vi "Configure Module.vi"(8 "error in (no error)":errorcluster, 10 "IOV ref in":refnum<k21>, 11 "Module Template in":refnum<class "9203.lvclass">) -> (0 "error out":errorcluster, 2 "IOV ref out":refnum<k21>, 3 "Module Template out":refnum<class "9203.lvclass">)   [LabVIEW 2011, in "Modules.lvlib" / "9203.lvclass"]
uses:
  9203.lvclass
  9203.lvclass/9203.ctl
  Program Files (x86)/National Instruments/LabVIEW 2011/resource/objmgr/cRIO.rc
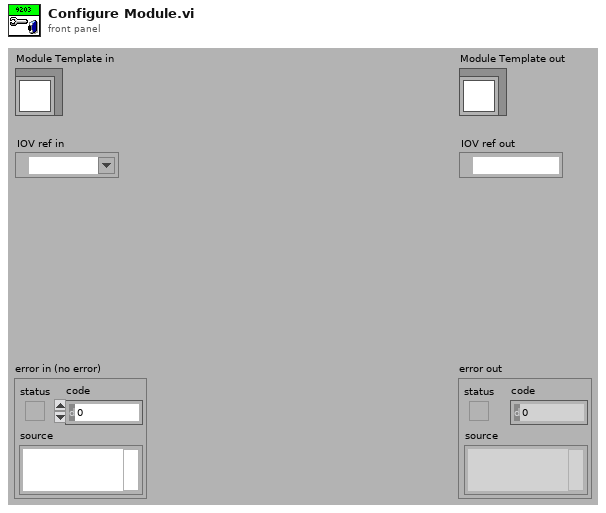
[diagram p1: front panel]
types:
  T1 = typedef "Modules.lvlib/9203.lvclass/Channel Settings.ctl" = cluster{"Range":T2}[]
  T2 = typedef "Modules.lvlib/9203.lvclass/Range.ctl" = u32
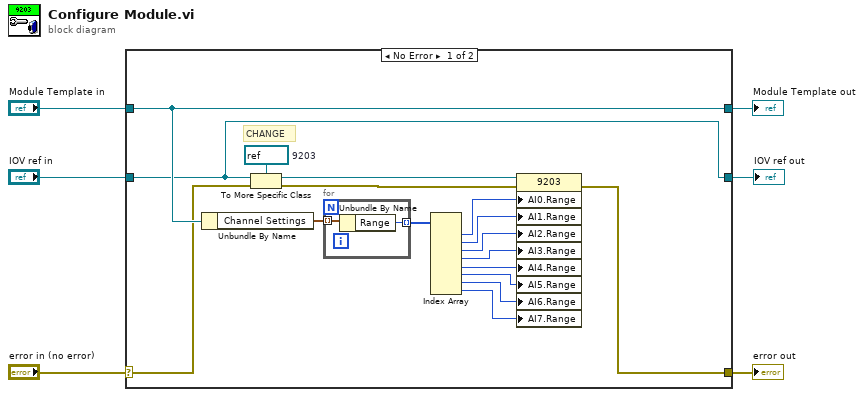
[diagram p0: block diagram]
diagram:
  n1 = case shown="No Error" "error in (no error)" {
    selector: "error in (no error)" -> [w22 w28]
    tunnel: [w18 w28] -> w5
    tunnel: [w23 w27] -> w3
    tunnel: "Module Template in" -> [w23 w27]
    tunnel: "IOV ref in" -> [w17 w26]
    tunnel: [w17 w26] -> w1
    frame No Error {
      w21 = refnum<k21> refnum  # 9203
      # "CHANGE"
      n2 = Unbundle By Name(w23) -> ("Channel Settings"=w16:T1)
      n3 = To More Specific Class(target class=w21, reference=w17, error in=w22) -> (specific class reference=w20:refnum<k21>, error out=w19:errorcluster)
      n4 = for {
        tunnel: w16 -> [w25] mode=indexing
        tunnel: [w24] -> w15 mode=indexing
        n5 = Unbundle By Name(w25) -> ("Range"=w24:T2)
      }
      n6 = Index Array(array=w15) -> (element #1=w14:T2, element #2=w13:T2, element #3=w12:T2, element #4=w11:T2, element #5=w10:T2, element #6=w9:T2, element #7=w8:T2, element #8=w7:T2)  [unwired: 8 in]
      n7 = property class="9203"(reference=w20, error in=w19, "AI0.Range"=w14, "AI1.Range"=w13, "AI2.Range"=w12, "AI3.Range"=w11, "AI4.Range"=w10, "AI5.Range"=w9, "AI6.Range"=w8, "AI7.Range"=w7) -> (error out=w18:errorcluster)  [unwired: 1 out]
    }
    frame Error {
    }
  }
  "error out" <- w5
  "Module Template out" <- w3
  "IOV ref out" <- w1
